vi "To Seconds From Midnight.vi"(8 "hour":i32, 9 "minute":i32, 10 "second":i32, 11 "fractional second":dbl) -> (3 "Numeric":dbl)   [LabVIEW 2020]
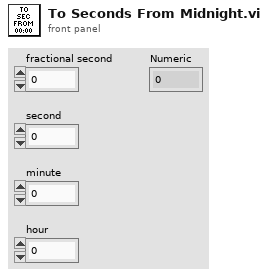
[diagram p1: front panel]
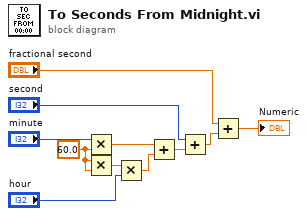
[diagram p0: block diagram]
diagram:
  w4 = 60.0 ("y")
  n1 = Multiply(x="minute", y=w4) -> (x*y=w6:dbl)
  n2 = Multiply(x=w4, y=w4) -> (x*y=w2:dbl)
  n3 = Multiply(x=w2, y="hour") -> (x*y=w5:dbl)
  n4 = Add(x=w6, y=w5) -> (x+y=w7:dbl)
  n5 = Add(x="second", y=w7) -> (x+y=w9:dbl)
  n6 = Add(x="fractional second", y=w9) -> (x+y=→"Numeric":dbl)
